vi "Edit Plugin Type Specialization - Single Converter.vi"(11 "error in":errorcluster) -> (15 "error out":errorcluster)   [LabVIEW 2021, in "Converter.lvlib"]
uses:
  Converter.lvlib
  Path Functions/Path Functions.lvlib
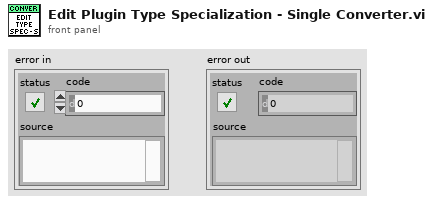
[diagram p1: front panel]
types:
  T1 = cluster{"parameter name":string, "type specialization":enum16{"none", "pin", "path", "enum"}, "annotations":cluster{"key":enum16{"none", "pin.instrument_type", "enum.values"}, "value":string}[]}[]
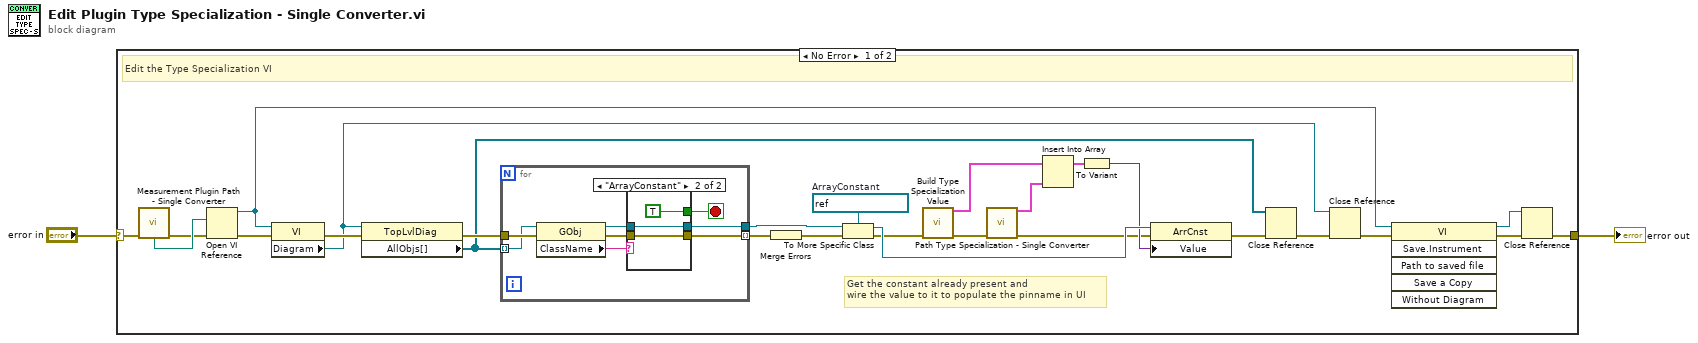
[diagram p0: block diagram]
diagram:
  n1 = case shown="No Error" "error in" {
    selector: "error in" -> [w9 w42]
    tunnel: [w4 w42] -> w1
    frame No Error {
      w21 = refnum<vi> refnum  # ArrayConstant
      # "Get the constant already present and\nwire the value to it to populate the pinname in UI"
      # "Edit the Type Specialization VI"
      n2 = call "Measurement Plugin Path - Single Converter.vi"("error in"=w9) -> ("type specialization"=w10:path, "error out"=w8:errorcluster)  [unwired: 2 in, 11 out]
      n3 = Open VI Reference(vi path=w10, error in (no error)=w8) -> (vi reference=w17:refnum<vi>, error out=w29:errorcluster)  [unwired: 4 in]
      n4 = property class="VI"(reference=w17, error in=w29) -> (error out=w28:errorcluster, "Diagram"=w23:refnum<vi>)  [unwired: 1 out]
      n5 = property class="TopLvlDiag"(reference=w23, error in=w28) -> (error out=w27:errorcluster, "AllObjs[]"=w24:refnum<vi>[])  [unwired: 1 out]
      n6 = for {
        tunnel: w24 -> [w36] mode=indexing
        tunnel: w27 -> [w37]
        tunnel: [w33] -> w22
        tunnel: [w31] -> w20 mode=indexing
        stop <- w32 stop-if-true
        n7 = property class="GObj"(reference=w36, error in=w37) -> (reference out=w34:refnum<vi>, error out=w35:errorcluster, "ClassName"=w30:string)
        n8 = case shown="\"ArrayConstant\"" w30 {
          tunnel: w35 -> [w38 w40]
          tunnel: w34 -> [_ w41]
          tunnel: [_ w41] -> w33
          tunnel: [_ TRUE] -> w32
          tunnel: [w38 w40] -> w31
          frame Default {
          }
          frame "ArrayConstant" {
          }
        }
      }
      n9 = Merge Errors(w20) -> (w19:errorcluster)
      n10 = To More Specific Class(target class=w21, reference=w22, error in=w19) -> (specific class reference=w16:refnum<vi>, error out=w15:errorcluster)
      n11 = call "Build Type Specialization Value.vi"("error in"=w15) -> ("type specialization"=w12:T1, "error out"=w6:errorcluster)  [unwired: 13 in]
      n12 = call "Path Type Specialization - Single Converter.vi"("error in"=w6) -> ("type specialization for path"=w7:T1, "error out"=w5:errorcluster)  [unwired: 13 in]
      n13 = Insert Into Array(array=w12, new element=w7) -> (w11:T1)  [unwired: 1 in]
      n14 = To Variant(anything=w11) -> (Variant=w14:variant)
      n15 = property class="ArrCnst"(reference=w16, error in=w5, "Value"=w14) -> (error out=w3:errorcluster)  [unwired: 1 out]
      n16 = Close Reference(reference=w24, error in (no error)=w3) -> (error out=w26:errorcluster)
      n17 = Close Reference(reference=w23, error in (no error)=w26) -> (error out=w25:errorcluster)
      n18 = invoke class="VI" method="Save.Instrument"(reference=w17, error in=w25) -> (reference out=w13:refnum<vi>, error out=w18:errorcluster)  [unwired: 4 in, 4 out]
      n19 = Close Reference(reference=w13, error in (no error)=w18) -> (error out=w4:errorcluster)
    }
    frame Error {
    }
  }
  "error out" <- w1
